vi "ALL arduinos connected 2.vi"() -> ()   [LabVIEW 2014]
uses:
  <vilib>/Utility/error.llb/DialogType.ctl
  <vilib>/Analysis/baseanly.llb/Mean (DBL).vi
  <vilib>/Instr/_visa.llb/VISA Configure Serial Port (Instr).vi
  <vilib>/Utility/file.llb/Write To Spreadsheet File (string).vi
  <vilib>/Utility/file.llb/Write To Spreadsheet File (DBL).vi
  <vilib>/Analysis/NI_AALBase.lvlib
panel:
  out "Input 6":string
  out "X 6":dbl format="%#_8g"
  out "x-y 6":dbl
  out "Y 6 7":dbl format="%#_8g"
  out "Waveform Chart 20":dbl[](graph) caption="Waveform Chart"
  out "Frequency 6":dbl format="%#_8g"
  out "Waveform Chart 19":dbl(graph) caption="Waveform Chart"
  out "Temperature 6":dbl
  out "Median 6":dbl format="%0.2f"
  out "Mean 6":dbl format="%0.2f"
  out "Waveform Chart 18":dbl(graph) caption="Waveform Chart"
  out "Input 5":string
  out "X 5":dbl format="%#_8g"
  out "x-y 5":dbl
  out "Y 5":dbl format="%#_8g"
  out "Waveform Chart 17":dbl[](graph) caption="Waveform Chart"
  out "Frequency 5":dbl format="%#_8g"
  out "Waveform Chart 16":dbl(graph) caption="Waveform Chart"
  out "Temperature 5":dbl
  out "Median 5":dbl format="%0.2f"
  out "Mean 5":dbl format="%0.2f"
  out "Waveform Chart 15":dbl(graph) caption="Waveform Chart"
  out "Input 4":string
  out "X 4":dbl format="%#_8g"
  out "x-y 4":dbl
  out "Y 4":dbl format="%#_8g"
  out "Waveform Chart 14":dbl[](graph) caption="Waveform Chart"
  out "Frequency 4":dbl format="%#_8g"
  out "Waveform Chart 6":dbl(graph) caption="Waveform Chart"
  out "Temperature 5":dbl
  out "Median 4":dbl format="%0.2f"
  out "Mean 4":dbl format="%0.2f"
  out "Waveform Chart 13":dbl(graph) caption="Waveform Chart"
  out "Input  3":string
  out "X 3":dbl format="%#_8g"
  out "x-y 3":dbl
  out "Y 3":dbl format="%#_8g"
  out "Waveform Chart 12":dbl[](graph) caption="Waveform Chart"
  out "Frequency 3":dbl format="%#_8g"
  out "Waveform Chart 5":dbl(graph) caption="Waveform Chart"
  out "Temperature 3":dbl
  out "Median 3":dbl format="%0.2f"
  out "Mean 3":dbl format="%0.2f"
  out "Waveform Chart 11":dbl(graph) caption="Waveform Chart"
  out "Input 1":string
  out "Input 2":string
  out "X 2":dbl format="%#_8g"
  out "x-y 2":dbl
  out "Y 2":dbl format="%#_8g"
  out "Waveform Chart 10":dbl[](graph) caption="Waveform Chart"
  out "Frequency 2":dbl format="%#_8g"
  out "Waveform Chart 4":dbl(graph) caption="Waveform Chart"
  out "Temperature 2":dbl
  out "Median 2":dbl format="%0.2f"
  out "Mean 2":dbl format="%0.2f"
  out "Waveform Chart 9":dbl(graph) caption="Waveform Chart"
  out "X 1 2":dbl format="%#_8g"
  out "x-y 1":dbl
  out "Y 1":dbl format="%#_8g"
  out "Waveform Chart 8":dbl[](graph) caption="Waveform Chart"
  out "Frequency 1":dbl format="%#_8g"
  out "Waveform Chart 3":dbl(graph) caption="Waveform Chart"
  out "Temperature 1":dbl
  out "Waveform Chart 7":dbl(graph) caption="Waveform Chart"
  out "Mean":dbl format="%0.2f"
  out "Median":dbl format="%0.2f"
  in  "STOP":bool
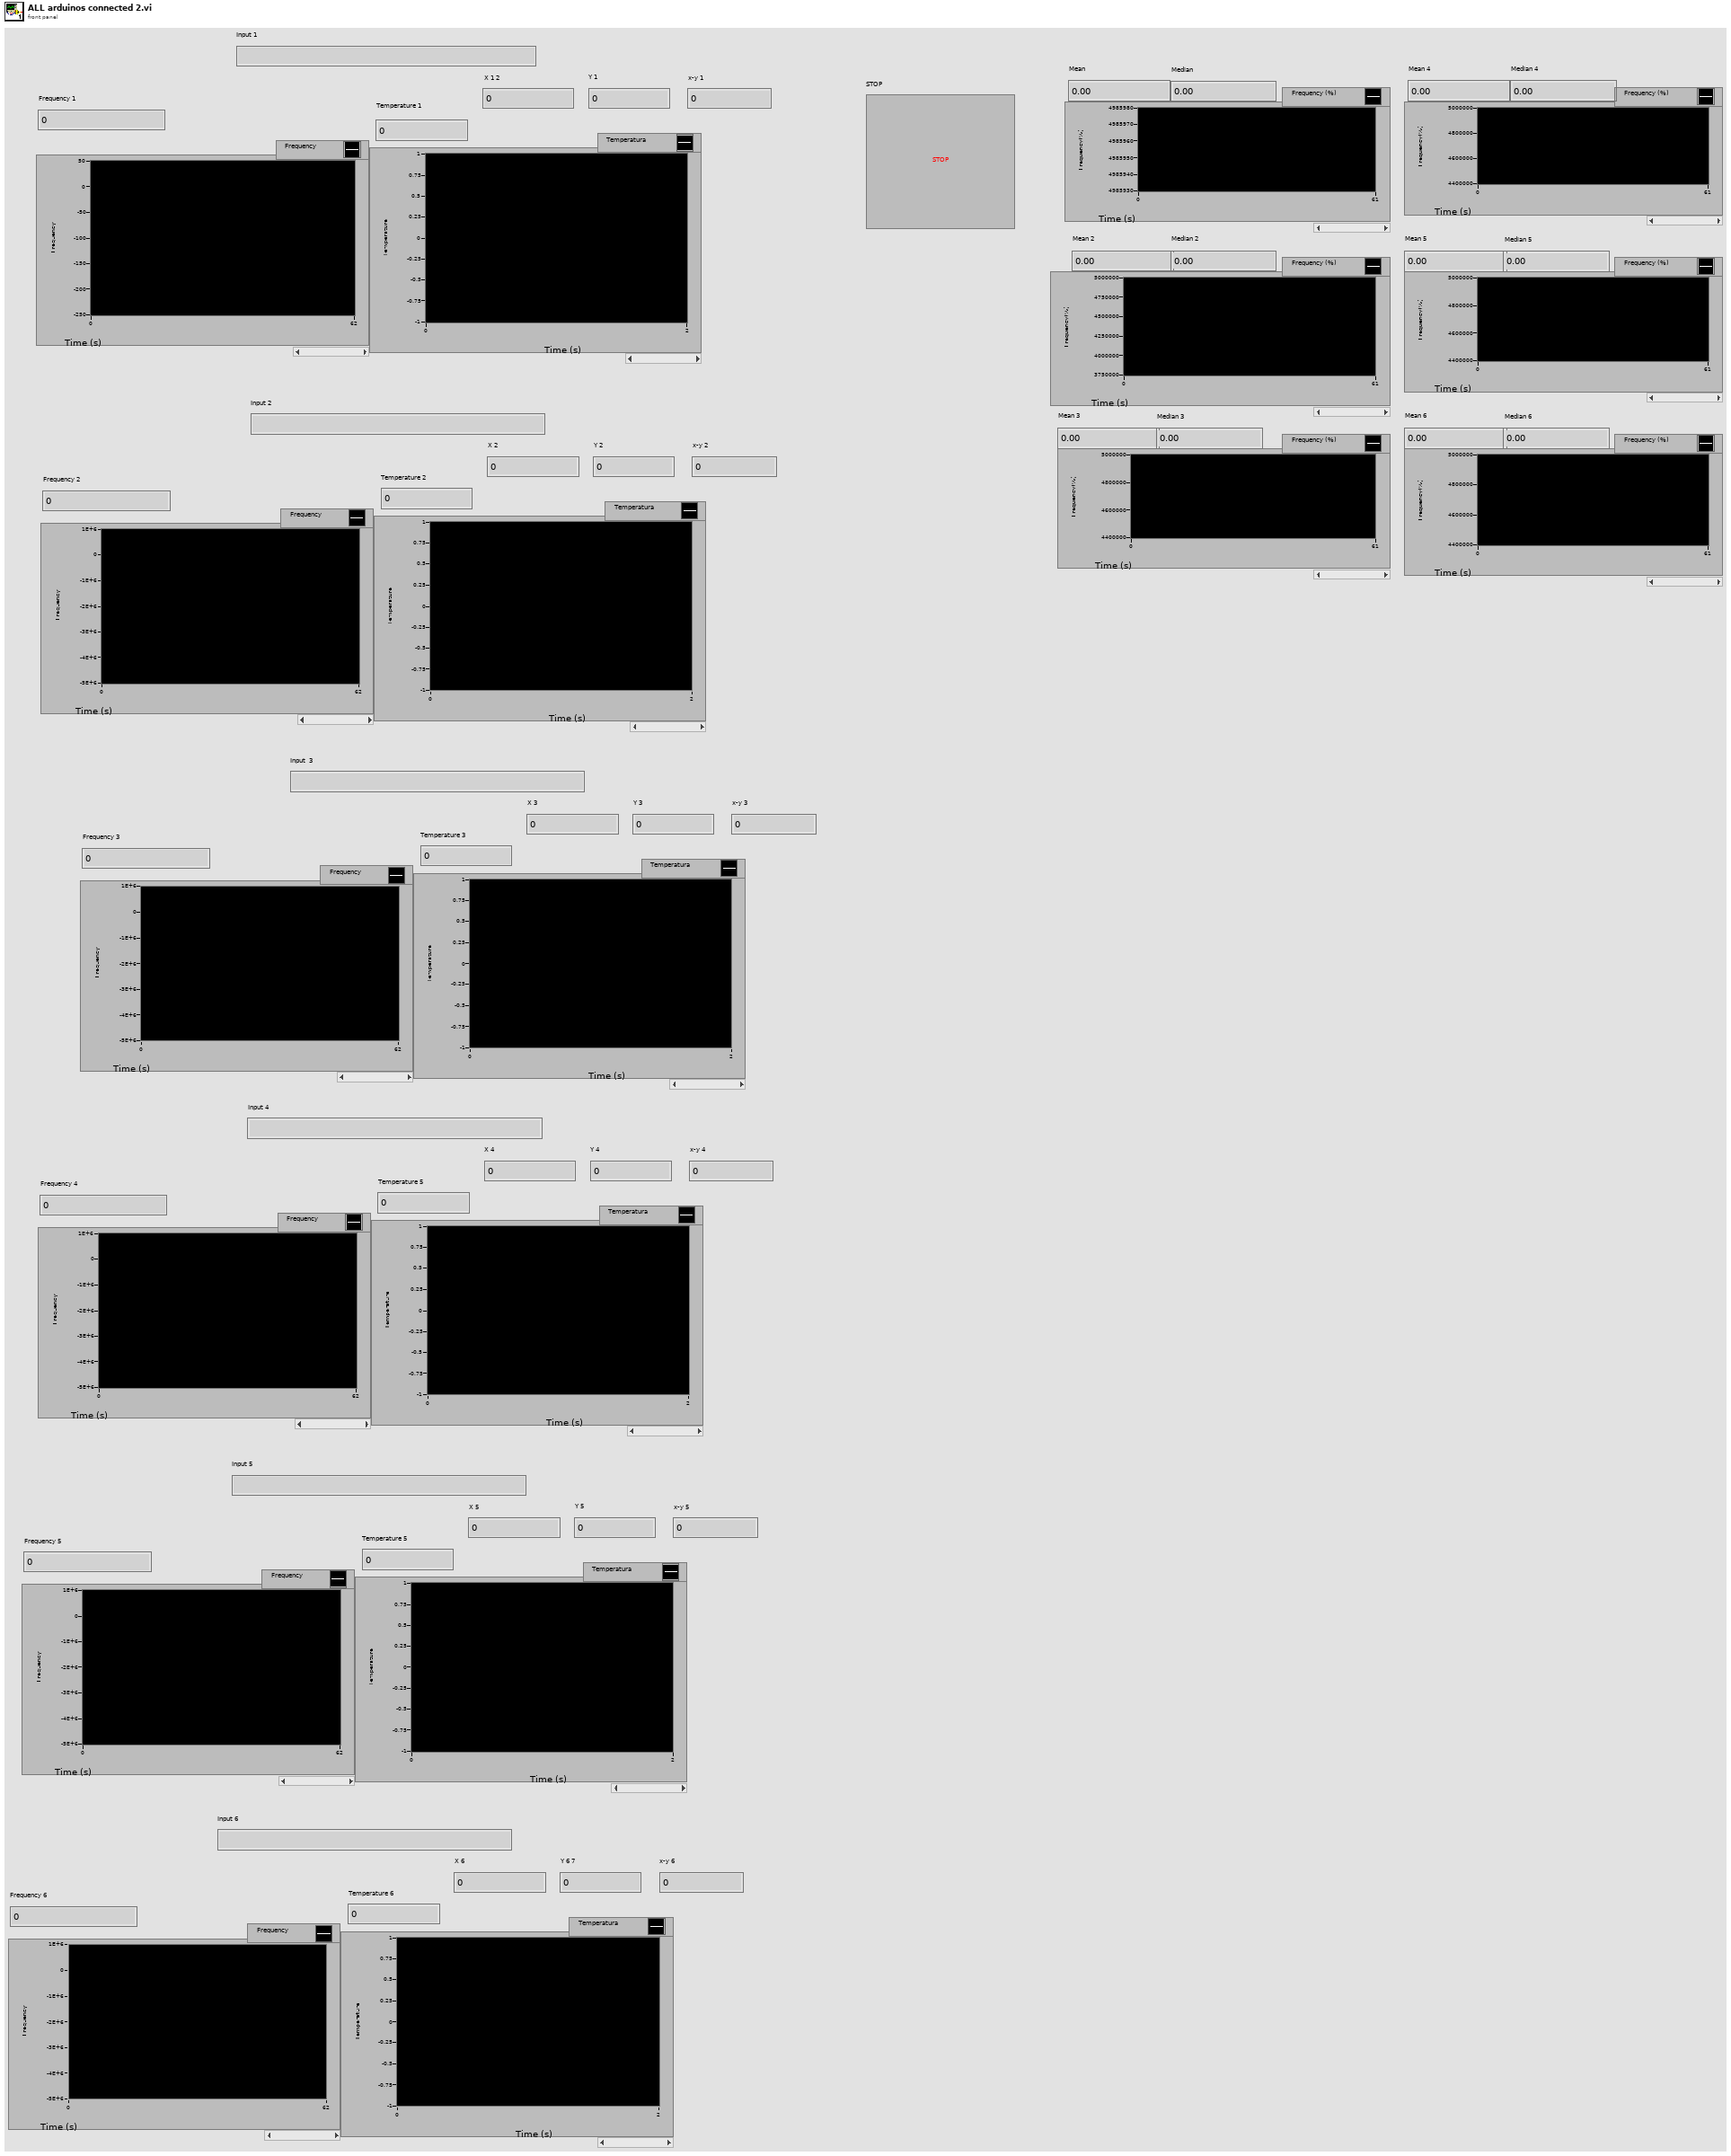
[diagram p1: front panel]
types:
  T1 = typedef "DialogType.ctl" = u16
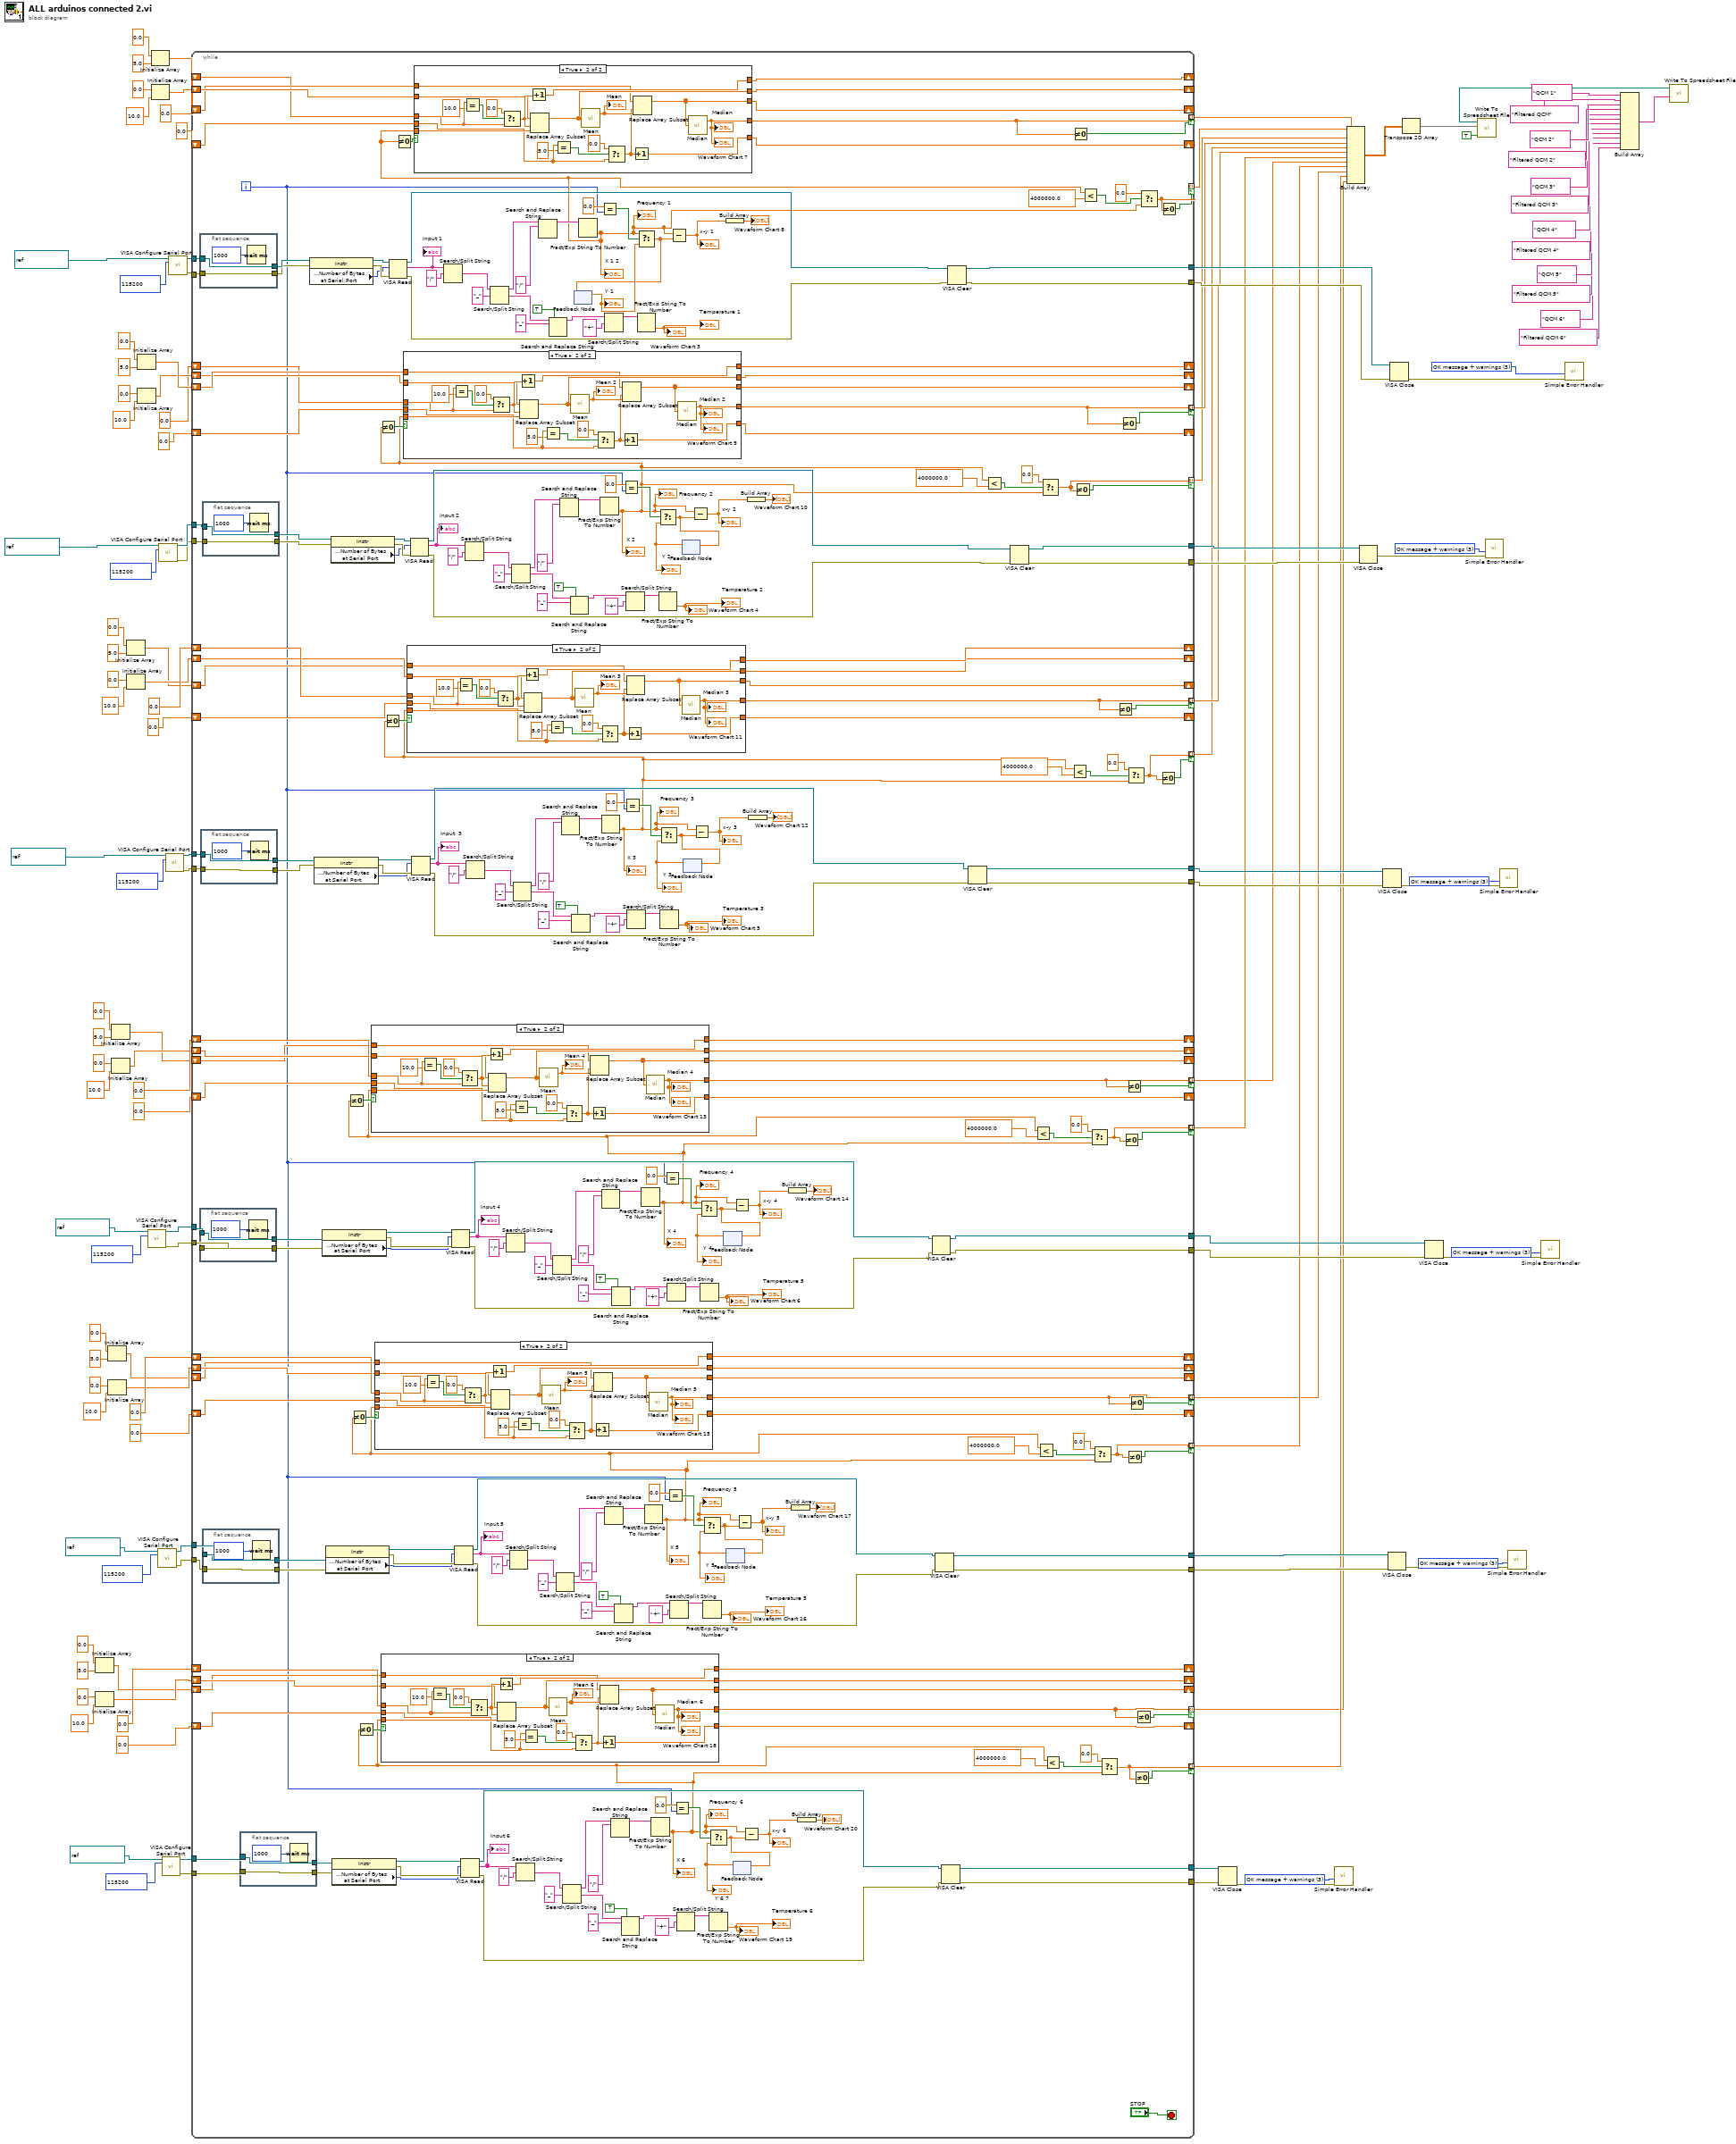
[diagram p0: block diagram]
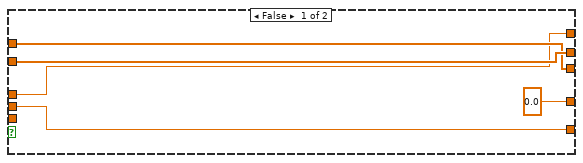
[diagram p2: hidden frame]
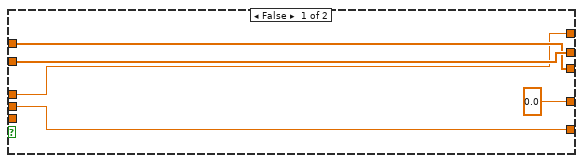
[diagram p3: hidden frame]
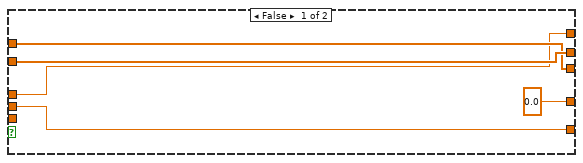
[diagram p4: hidden frame]
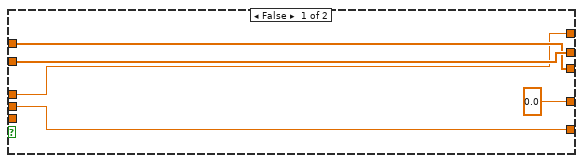
[diagram p5: hidden frame]
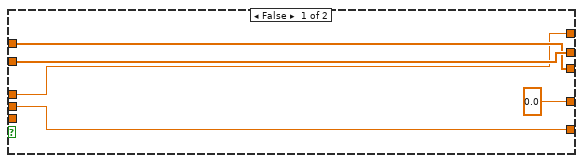
[diagram p6: hidden frame]
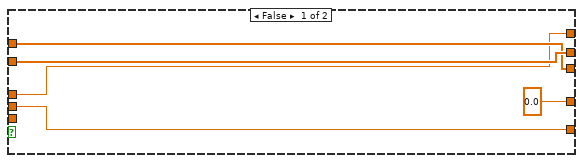
[diagram p7: hidden frame]
diagram:
  w6 = T1 3 items=["no dialog", "OK message", "continue or stop message", "OK message + warnings", "continue/stop + warnings"] ("type of dialog (OK msg:1)")
  w32 = T1 3 items=["no dialog", "OK message", "continue or stop message", "OK message + warnings", "continue/stop + warnings"] ("type of dialog (OK msg:1)")
  w48 = T1 3 items=["no dialog", "OK message", "continue or stop message", "OK message + warnings", "continue/stop + warnings"] ("type of dialog (OK msg:1)")
  w67 = T1 3 items=["no dialog", "OK message", "continue or stop message", "OK message + warnings", "continue/stop + warnings"] ("type of dialog (OK msg:1)")
  w90 = T1 3 items=["no dialog", "OK message", "continue or stop message", "OK message + warnings", "continue/stop + warnings"] ("type of dialog (OK msg:1)")
  w106 = T1 3 items=["no dialog", "OK message", "continue or stop message", "OK message + warnings", "continue/stop + warnings"] ("type of dialog (OK msg:1)")
  n1 = Initialize Array(0.0 ("x"), 5.0 ("x")) -> (w12:dbl[])
  n2 = Initialize Array(0.0 ("x"), 10.0 ("x")) -> (w13:dbl[])
  n3 = Initialize Array(0.0 ("x"), 5.0 ("x")) -> (w34:dbl[])
  n4 = Initialize Array(0.0 ("x"), 10.0 ("x")) -> (w35:dbl[])
  n5 = Initialize Array(0.0 ("x"), 5.0 ("x")) -> (w54:dbl[])
  n6 = Initialize Array(0.0 ("x"), 10.0 ("x")) -> (w55:dbl[])
  n7 = Initialize Array(0.0 ("x"), 5.0 ("x")) -> (w73:dbl[])
  n8 = Initialize Array(0.0 ("x"), 10.0 ("x")) -> (w74:dbl[])
  n9 = Initialize Array(0.0 ("x"), 5.0 ("x")) -> (w83:dbl[])
  n10 = Initialize Array(0.0 ("x"), 10.0 ("x")) -> (w82:dbl[])
  n11 = call-poly "VISA Configure Serial Port"("VISA resource name"=refnum<visa-resource-name> "COM12", "baud rate (9600)"=u32 115200) -> ("VISA resource name out"=w50:refnum<visa-resource-name>, "error out"=w49:errorcluster)  [unwired: 12 in]
  n12 = Initialize Array(0.0 ("x"), 5.0 ("x")) -> (w115:dbl[])
  n13 = Initialize Array(0.0 ("x"), 10.0 ("x")) -> (w119:dbl[])
  n14 = call-poly "VISA Configure Serial Port"("VISA resource name"=refnum<visa-resource-name> "COM12", "baud rate (9600)"=u32 115200) -> ("VISA resource name out"=w20:refnum<visa-resource-name>, "error out"=w19:errorcluster)  [unwired: 12 in]
  n15 = call-poly "VISA Configure Serial Port"("VISA resource name"=refnum<visa-resource-name> "COM12", "baud rate (9600)"=u32 115200) -> ("VISA resource name out"=w92:refnum<visa-resource-name>, "error out"=w91:errorcluster)  [unwired: 12 in]
  n16 = call-poly "VISA Configure Serial Port"("VISA resource name"=refnum<visa-resource-name> "COM12", "baud rate (9600)"=u32 115200) -> ("VISA resource name out"=w8:refnum<visa-resource-name>, "error out"=w7:errorcluster)  [unwired: 12 in]
  n17 = call-poly "VISA Configure Serial Port"("VISA resource name"=refnum<visa-resource-name> "COM12", "baud rate (9600)"=u32 115200) -> ("VISA resource name out"=w69:refnum<visa-resource-name>, "error out"=w68:errorcluster)  [unwired: 12 in]
  n18 = call-poly "VISA Configure Serial Port"("VISA resource name"=refnum<visa-resource-name> "COM10", "baud rate (9600)"=u32 115200) -> ("VISA resource name out"=w108:refnum<visa-resource-name>, "error out"=w107:errorcluster)  [unwired: 12 in]
  n19 = while {
    shift-right: [w369] -> _
    shift-left: w119 -> [w414]
    shift-right: [w368] -> _
    shift-left: 0.0 ("x") -> [w327]
    shift-right: [w412] -> _
    shift-left: w115 -> [w411]
    shift-right: [w410] -> _
    shift-left: 0.0 ("x") -> [w409]
    tunnel: [w407] -> w85 mode=indexing if=w408
    tunnel: w108 -> [w406]
    tunnel: w107 -> [w405]
    tunnel: [w377] -> w104
    tunnel: [w376] -> w103
    tunnel: [w372] -> w86 mode=indexing if=w371
    tunnel: [w366] -> w84 mode=indexing if=w367
    tunnel: w92 -> [w339]
    tunnel: w91 -> [w338]
    tunnel: [w333] -> w88
    tunnel: [w332] -> w87
    tunnel: [w331] -> w63 mode=indexing if=w330
    shift-right: [w326] -> _
    shift-left: w83 -> [w325]
    shift-right: [w323] -> _
    shift-left: w82 -> [w324]
    shift-right: [w321] -> _
    shift-left: 0.0 ("x") -> [w322]
    shift-right: [w319] -> _
    shift-left: 0.0 ("x") -> [w320]
    tunnel: [w308] -> w62 mode=indexing if=w309
    shift-right: [w313] -> _
    shift-left: 0.0 ("x") -> [w317]
    shift-right: [w312] -> _
    shift-left: w74 -> [w316]
    shift-right: [w311] -> _
    shift-left: w73 -> [w315]
    shift-right: [w310] -> _
    shift-left: 0.0 ("x") -> [w314]
    tunnel: w69 -> [w307]
    tunnel: w68 -> [w306]
    tunnel: [w278] -> w65
    tunnel: [w277] -> w64
    tunnel: [w272] -> w61 mode=indexing if=w271
    tunnel: w50 -> [w265]
    tunnel: w49 -> [w264]
    tunnel: [w236] -> w46
    tunnel: [w235] -> w45
    tunnel: [w231] -> w42 mode=indexing if=w230
    shift-right: [w228] -> _
    shift-left: 0.0 ("x") -> [w269]
    shift-right: [w227] -> _
    shift-left: w55 -> [w268]
    shift-right: [w226] -> _
    shift-left: w54 -> [w267]
    tunnel: [w224] -> w41 mode=indexing if=w225
    shift-right: [w223] -> _
    shift-left: 0.0 ("x") -> [w266]
    tunnel: [w186] -> w26 mode=indexing if=w185
    tunnel: [w181] -> w25 mode=indexing if=w180
    shift-right: [w184] -> _
    shift-left: 0.0 ("x") -> [w190]
    shift-right: [w183] -> _
    shift-left: w35 -> [w189]
    shift-right: [w182] -> _
    shift-left: w34 -> [w188]
    shift-right: [w179] -> _
    shift-left: 0.0 ("x") -> [w187]
    tunnel: [w178] -> w30
    tunnel: [w177] -> w29
    tunnel: w20 -> [w145]
    tunnel: w19 -> [w144]
    tunnel: w8 -> [w138]
    tunnel: w7 -> [w137]
    tunnel: [w132] -> w1 mode=indexing if=w131
    tunnel: [w129] -> w2 mode=indexing if=w128
    tunnel: [w127] -> w4
    tunnel: [w126] -> w3
    shift-right: [w135] -> _
    shift-left: 0.0 ("x") -> [w143]
    shift-right: [w134] -> _
    shift-left: w13 -> [w142]
    shift-right: [w133] -> _
    shift-left: w12 -> [w141]
    shift-right: [w130] -> _
    shift-left: 0.0 ("x") -> [w140]
    i -> [w139]
    stop <- "STOP" stop-if-true
    n20 = flat-sequence {
      tunnel: [w471] -> w262
      tunnel: w265 -> [w471]
      tunnel: w264 -> [w470]
      tunnel: [w470] -> w263
      frame #0 {
        n21 = Wait (ms)(milliseconds to wait=u32 1000) -> ()  [unwired: 1 out]
      }
    }
    n22 = flat-sequence {
      tunnel: [w552] -> w381
      tunnel: w406 -> [w552]
      tunnel: w405 -> [w551]
      tunnel: [w551] -> w380
      frame #0 {
        n23 = Wait (ms)(milliseconds to wait=u32 1000) -> ()  [unwired: 1 out]
      }
    }
    n24 = flat-sequence {
      tunnel: [w498] -> w282
      tunnel: w307 -> [w498]
      tunnel: w306 -> [w497]
      tunnel: [w497] -> w281
      frame #0 {
        n25 = Wait (ms)(milliseconds to wait=u32 1000) -> ()  [unwired: 1 out]
      }
    }
    n26 = flat-sequence {
      tunnel: [w525] -> w337
      tunnel: w339 -> [w525]
      tunnel: w338 -> [w524]
      tunnel: [w524] -> w336
      frame #0 {
        n27 = Wait (ms)(milliseconds to wait=u32 1000) -> ()  [unwired: 1 out]
      }
    }
    n28 = flat-sequence {
      tunnel: [w444] -> w220
      tunnel: w145 -> [w444]
      tunnel: w144 -> [w443]
      tunnel: [w443] -> w221
      frame #0 {
        n29 = Wait (ms)(milliseconds to wait=u32 1000) -> ()  [unwired: 1 out]
      }
    }
    n30 = flat-sequence {
      tunnel: [w417] -> w174
      tunnel: w138 -> [w417]
      tunnel: w137 -> [w416]
      tunnel: [w416] -> w175
      frame #0 {
        n31 = Wait (ms)(milliseconds to wait=u32 1000) -> ()  [unwired: 1 out]
      }
    }
    n32 = property class="Instr"(reference=w381, error in=w380) -> (reference out=w385:refnum<visa-resource-name>, error out=w384:errorcluster, "Serial Settings:Number of Bytes at Serial Port"=w383:u32)
    n33 = property class="Instr"(reference=w282, error in=w281) -> (reference out=w286:refnum<visa-resource-name>, error out=w285:errorcluster, "Serial Settings:Number of Bytes at Serial Port"=w284:u32)
    n34 = property class="Instr"(reference=w262, error in=w263) -> (reference out=w241:refnum<visa-resource-name>, error out=w240:errorcluster, "Serial Settings:Number of Bytes at Serial Port"=w239:u32)
    n35 = property class="Instr"(reference=w220, error in=w221) -> (reference out=w199:refnum<visa-resource-name>, error out=w198:errorcluster, "Serial Settings:Number of Bytes at Serial Port"=w197:u32)
    n36 = property class="Instr"(reference=w337, error in=w336) -> (reference out=w343:refnum<visa-resource-name>, error out=w342:errorcluster, "Serial Settings:Number of Bytes at Serial Port"=w341:u32)
    n37 = property class="Instr"(reference=w174, error in=w175) -> (reference out=w153:refnum<visa-resource-name>, error out=w152:errorcluster, "Serial Settings:Number of Bytes at Serial Port"=w151:u32)
    n38 = VISA Read(VISA resource name=w385, byte count=w383, error in (no error)=w384) -> (VISA resource name out=w378:refnum<visa-resource-name>, read buffer=w386:string, error out=w379:errorcluster)  [unwired: 1 out]
    "Input 1" <- w386
    n39 = VISA Read(VISA resource name=w343, byte count=w341, error in (no error)=w342) -> (VISA resource name out=w335:refnum<visa-resource-name>, read buffer=w344:string, error out=w334:errorcluster)  [unwired: 1 out]
    "Input 2" <- w344
    n40 = VISA Read(VISA resource name=w286, byte count=w284, error in (no error)=w285) -> (VISA resource name out=w280:refnum<visa-resource-name>, read buffer=w287:string, error out=w279:errorcluster)  [unwired: 1 out]
    "Input  3" <- w287
    n41 = Search/Split String(string=w386, search string/char (-)="/") -> (match + rest of string=w395:string)  [unwired: 1 in, 2 out]
    n42 = VISA Read(VISA resource name=w241, byte count=w239, error in (no error)=w240) -> (VISA resource name out=w238:refnum<visa-resource-name>, read buffer=w243:string, error out=w237:errorcluster)  [unwired: 1 out]
    "Input 4" <- w243
    n43 = VISA Read(VISA resource name=w199, byte count=w197, error in (no error)=w198) -> (VISA resource name out=w196:refnum<visa-resource-name>, read buffer=w201:string, error out=w195:errorcluster)  [unwired: 1 out]
    "Input 5" <- w201
    n44 = VISA Read(VISA resource name=w153, byte count=w151, error in (no error)=w152) -> (VISA resource name out=w150:refnum<visa-resource-name>, read buffer=w155:string, error out=w136:errorcluster)  [unwired: 1 out]
    "Input 6" <- w155
    n45 = Search/Split String(string=w344, search string/char (-)="/") -> (match + rest of string=w353:string)  [unwired: 1 in, 2 out]
    n46 = Search/Split String(string=w287, search string/char (-)="/") -> (match + rest of string=w296:string)  [unwired: 1 in, 2 out]
    n47 = Search/Split String(string=w395, search string/char (-)="_") -> (substring before match=w388:string, match + rest of string=w394:string)  [unwired: 1 in, 1 out]
    n48 = Search/Split String(string=w243, search string/char (-)="/") -> (match + rest of string=w252:string)  [unwired: 1 in, 2 out]
    n49 = Search/Split String(string=w201, search string/char (-)="/") -> (match + rest of string=w210:string)  [unwired: 1 in, 2 out]
    n50 = Search/Split String(string=w353, search string/char (-)="_") -> (substring before match=w346:string, match + rest of string=w352:string)  [unwired: 1 in, 1 out]
    n51 = Search/Split String(string=w296, search string/char (-)="_") -> (substring before match=w289:string, match + rest of string=w295:string)  [unwired: 1 in, 1 out]
    n52 = Search/Split String(string=w155, search string/char (-)="/") -> (match + rest of string=w164:string)  [unwired: 1 in, 2 out]
    n53 = Search and Replace String(input string=w388, search string="/" ("replace string (\"\")")) -> (result string=w398:string)  [unwired: 6 in, 3 out]
    n54 = Search and Replace String(replace all?=TRUE ("replace all? (F)"), input string=w394, search string="_") -> (result string=w390:string)  [unwired: 5 in, 3 out]
    n55 = Search/Split String(string=w252, search string/char (-)="_") -> (substring before match=w245:string, match + rest of string=w251:string)  [unwired: 1 in, 1 out]
    n56 = Search/Split String(string=w210, search string/char (-)="_") -> (substring before match=w203:string, match + rest of string=w209:string)  [unwired: 1 in, 1 out]
    n57 = Search and Replace String(input string=w346, search string="/" ("replace string (\"\")")) -> (result string=w356:string)  [unwired: 6 in, 3 out]
    n58 = Search and Replace String(input string=w289, search string="/" ("replace string (\"\")")) -> (result string=w299:string)  [unwired: 6 in, 3 out]
    n59 = Search/Split String(string=w164, search string/char (-)="_") -> (substring before match=w157:string, match + rest of string=w163:string)  [unwired: 1 in, 1 out]
    n60 = Search and Replace String(replace all?=TRUE ("replace all? (F)"), input string=w352, search string="_") -> (result string=w348:string)  [unwired: 5 in, 3 out]
    n61 = Search and Replace String(replace all?=TRUE ("replace all? (F)"), input string=w295, search string="_") -> (result string=w291:string)  [unwired: 5 in, 3 out]
    n62 = feedback #1() -> (w402:dbl)  [unwired: 1 in]
    "Y 1" <- w402
    n63 = Fract/Exp String To Number(string=w398) -> (number=w370:dbl)  [unwired: 3 in, 1 out]
    "Frequency 1" <- w370
    "X 1 2" <- w370
    n64 = Not Equal To 0?(x=w370) -> (x != 0?=w413:bool)
    n65 = case shown="True" w413 {
      tunnel: w414 -> [w558 w571]
      tunnel: w327 -> [w555 w574]
      tunnel: [w555 w573] -> w368
      tunnel: w370 -> [_ w572]
      tunnel: [w558 w570] -> w369
      tunnel: [w557 w562] -> w412
      tunnel: w411 -> [w557 w563]
      tunnel: w409 -> [w556 w566]
      tunnel: [w556 w564] -> w410
      tunnel: [0.0 ("median") w559] -> w407
      frame False {
      }
      frame True {
        n66 = Equal?(x=w574, y=10.0) -> (x = y?=w577:bool)
        n67 = Select(t=0.0, s=w577, f=w574) -> (s? t:f=w575:dbl)
        n68 = Increment(x=w575) -> (x+1=w573:dbl)
        n69 = Replace Array Subset(array=w571, new element=w572, index=w575) -> (w570:dbl[])
        n70 = Equal?(x=w566, y=5.0) -> (x = y?=w567:bool)
        n71 = call-poly <vilib>:"Mean.vi"("X"=w570) -> ("mean"=w569:dbl)  [unwired: 1 out]
        "Mean" <- w569
        n72 = Select(t=0.0, s=w567, f=w566) -> (s? t:f=w565:dbl)
        n73 = Increment(x=w565) -> (x+1=w564:dbl)
        n74 = Replace Array Subset(array=w563, new element=w569, index=w565) -> (w562:dbl[])
        n75 = call <vilib>:"Median.vi"("X"=w562) -> ("median"=w559:dbl)  [unwired: 1 out]
        "Median" <- w559
        "Waveform Chart 7" <- w559
      }
    }
    n76 = Fract/Exp String To Number(string=w356) -> (number=w328:dbl)  [unwired: 3 in, 1 out]
    "Frequency 2" <- w328
    "X 2" <- w328
    n77 = Not Equal To 0?(x=w328) -> (x != 0?=w329:bool)
    n78 = case shown="True" w329 {
      tunnel: w324 -> [w531 w544]
      tunnel: w322 -> [w528 w547]
      tunnel: [w528 w546] -> w321
      tunnel: w328 -> [_ w545]
      tunnel: [w531 w543] -> w323
      tunnel: [w530 w535] -> w326
      tunnel: w325 -> [w530 w536]
      tunnel: w320 -> [w529 w539]
      tunnel: [w529 w537] -> w319
      tunnel: [0.0 ("median") w532] -> w366
      frame False {
      }
      frame True {
        n79 = Equal?(x=w547, y=10.0) -> (x = y?=w550:bool)
        n80 = Select(t=0.0, s=w550, f=w547) -> (s? t:f=w548:dbl)
        n81 = Increment(x=w548) -> (x+1=w546:dbl)
        n82 = Replace Array Subset(array=w544, new element=w545, index=w548) -> (w543:dbl[])
        n83 = Equal?(x=w539, y=5.0) -> (x = y?=w540:bool)
        n84 = call-poly <vilib>:"Mean.vi"("X"=w543) -> ("mean"=w542:dbl)  [unwired: 1 out]
        "Mean 2" <- w542
        n85 = Select(t=0.0, s=w540, f=w539) -> (s? t:f=w538:dbl)
        n86 = Increment(x=w538) -> (x+1=w537:dbl)
        n87 = Replace Array Subset(array=w536, new element=w542, index=w538) -> (w535:dbl[])
        n88 = call <vilib>:"Median.vi"("X"=w535) -> ("median"=w532:dbl)  [unwired: 1 out]
        "Median 2" <- w532
        "Waveform Chart 9" <- w532
      }
    }
    n89 = Equal?(x=0.0, y=w139) -> (x = y?=w403:bool)
    n90 = Fract/Exp String To Number(string=w299) -> (number=w273:dbl)  [unwired: 3 in, 1 out]
    "Frequency 3" <- w273
    "X 3" <- w273
    n91 = Not Equal To 0?(x=w273) -> (x != 0?=w318:bool)
    n92 = case shown="True" w318 {
      tunnel: w316 -> [w504 w517]
      tunnel: w317 -> [w501 w520]
      tunnel: [w501 w519] -> w313
      tunnel: w273 -> [_ w518]
      tunnel: [w504 w516] -> w312
      tunnel: [w503 w508] -> w311
      tunnel: w315 -> [w503 w509]
      tunnel: w314 -> [w502 w512]
      tunnel: [w502 w510] -> w310
      tunnel: [0.0 ("median") w505] -> w308
      frame False {
      }
      frame True {
        n93 = Equal?(x=w520, y=10.0) -> (x = y?=w523:bool)
        n94 = Select(t=0.0, s=w523, f=w520) -> (s? t:f=w521:dbl)
        n95 = Increment(x=w521) -> (x+1=w519:dbl)
        n96 = Replace Array Subset(array=w517, new element=w518, index=w521) -> (w516:dbl[])
        n97 = Equal?(x=w512, y=5.0) -> (x = y?=w513:bool)
        n98 = call-poly <vilib>:"Mean.vi"("X"=w516) -> ("mean"=w515:dbl)  [unwired: 1 out]
        "Mean 3" <- w515
        n99 = Select(t=0.0, s=w513, f=w512) -> (s? t:f=w511:dbl)
        n100 = Increment(x=w511) -> (x+1=w510:dbl)
        n101 = Replace Array Subset(array=w509, new element=w515, index=w511) -> (w508:dbl[])
        n102 = call <vilib>:"Median.vi"("X"=w508) -> ("median"=w505:dbl)  [unwired: 1 out]
        "Median 3" <- w505
        "Waveform Chart 11" <- w505
      }
    }
    n103 = Search and Replace String(input string=w245, search string="/" ("replace string (\"\")")) -> (result string=w255:string)  [unwired: 6 in, 3 out]
    n104 = Search/Split String(string=w390, search string/char (-)="+") -> (substring before match=w391:string)  [unwired: 1 in, 2 out]
    n105 = Search and Replace String(input string=w203, search string="/" ("replace string (\"\")")) -> (result string=w213:string)  [unwired: 6 in, 3 out]
    n106 = Search and Replace String(input string=w157, search string="/" ("replace string (\"\")")) -> (result string=w167:string)  [unwired: 6 in, 3 out]
    n107 = Search and Replace String(replace all?=TRUE ("replace all? (F)"), input string=w251, search string="_") -> (result string=w247:string)  [unwired: 5 in, 3 out]
    n108 = Search and Replace String(replace all?=TRUE ("replace all? (F)"), input string=w209, search string="_") -> (result string=w205:string)  [unwired: 5 in, 3 out]
    n109 = Search and Replace String(replace all?=TRUE ("replace all? (F)"), input string=w163, search string="_") -> (result string=w159:string)  [unwired: 5 in, 3 out]
    n110 = Equal?(x=0.0, y=w139) -> (x = y?=w361:bool)
    n111 = Equal?(x=0.0, y=w139) -> (x = y?=w304:bool)
    n112 = Search/Split String(string=w348, search string/char (-)="+") -> (substring before match=w349:string)  [unwired: 1 in, 2 out]
    n113 = Search/Split String(string=w291, search string/char (-)="+") -> (substring before match=w292:string)  [unwired: 1 in, 2 out]
    n114 = Select(t=w370, s=w403, f=w402) -> (s? t:f=w401:dbl)
    n115 = feedback-in #1(w401) -> ()
    n116 = Fract/Exp String To Number(string=w391) -> (number=→"Temperature 1" →"Waveform Chart 3":dbl)  [unwired: 3 in, 1 out]
    n117 = Fract/Exp String To Number(string=w255) -> (number=w229:dbl)  [unwired: 3 in, 1 out]
    "Frequency 4" <- w229
    "X 4" <- w229
    n118 = Not Equal To 0?(x=w229) -> (x != 0?=w270:bool)
    n119 = case shown="True" w270 {
      tunnel: w268 -> [w477 w490]
      tunnel: w269 -> [w474 w493]
      tunnel: [w474 w492] -> w228
      tunnel: w229 -> [_ w491]
      tunnel: [w477 w489] -> w227
      tunnel: [w476 w482] -> w226
      tunnel: w267 -> [w476 w483]
      tunnel: w266 -> [w475 w478]
      tunnel: [w475 w484] -> w223
      tunnel: [0.0 ("median") w479] -> w224
      frame False {
      }
      frame True {
        n120 = Equal?(x=w493, y=10.0) -> (x = y?=w496:bool)
        n121 = Select(t=0.0, s=w496, f=w493) -> (s? t:f=w494:dbl)
        n122 = Increment(x=w494) -> (x+1=w492:dbl)
        n123 = Replace Array Subset(array=w490, new element=w491, index=w494) -> (w489:dbl[])
        n124 = Equal?(x=w478, y=5.0) -> (x = y?=w486:bool)
        n125 = call-poly <vilib>:"Mean.vi"("X"=w489) -> ("mean"=w488:dbl)  [unwired: 1 out]
        "Mean 4" <- w488
        n126 = Select(t=0.0, s=w486, f=w478) -> (s? t:f=w485:dbl)
        n127 = Increment(x=w485) -> (x+1=w484:dbl)
        n128 = Replace Array Subset(array=w483, new element=w488, index=w485) -> (w482:dbl[])
        n129 = call <vilib>:"Median.vi"("X"=w482) -> ("median"=w479:dbl)  [unwired: 1 out]
        "Median 4" <- w479
        "Waveform Chart 13" <- w479
      }
    }
    n130 = Fract/Exp String To Number(string=w213) -> (number=w191:dbl)  [unwired: 3 in, 1 out]
    "Frequency 5" <- w191
    "X 5" <- w191
    n131 = Not Equal To 0?(x=w191) -> (x != 0?=w222:bool)
    n132 = case shown="True" w222 {
      tunnel: w189 -> [w450 w463]
      tunnel: w190 -> [w447 w466]
      tunnel: [w447 w465] -> w184
      tunnel: w191 -> [_ w464]
      tunnel: [w450 w462] -> w183
      tunnel: [w449 w455] -> w182
      tunnel: w188 -> [w449 w456]
      tunnel: w187 -> [w448 w451]
      tunnel: [w448 w457] -> w179
      tunnel: [0.0 ("median") w452] -> w181
      frame False {
      }
      frame True {
        n133 = Equal?(x=w466, y=10.0) -> (x = y?=w469:bool)
        n134 = Select(t=0.0, s=w469, f=w466) -> (s? t:f=w467:dbl)
        n135 = Increment(x=w467) -> (x+1=w465:dbl)
        n136 = Replace Array Subset(array=w463, new element=w464, index=w467) -> (w462:dbl[])
        n137 = Equal?(x=w451, y=5.0) -> (x = y?=w459:bool)
        n138 = call-poly <vilib>:"Mean.vi"("X"=w462) -> ("mean"=w461:dbl)  [unwired: 1 out]
        "Mean 5" <- w461
        n139 = Select(t=0.0, s=w459, f=w451) -> (s? t:f=w458:dbl)
        n140 = Increment(x=w458) -> (x+1=w457:dbl)
        n141 = Replace Array Subset(array=w456, new element=w461, index=w458) -> (w455:dbl[])
        n142 = call <vilib>:"Median.vi"("X"=w455) -> ("median"=w452:dbl)  [unwired: 1 out]
        "Median 5" <- w452
        "Waveform Chart 15" <- w452
      }
    }
    n143 = Fract/Exp String To Number(string=w167) -> (number=w146:dbl)  [unwired: 3 in, 1 out]
    "Frequency 6" <- w146
    "X 6" <- w146
    n144 = Not Equal To 0?(x=w146) -> (x != 0?=w176:bool)
    n145 = case shown="True" w176 {
      tunnel: w142 -> [w423 w436]
      tunnel: w143 -> [w420 w439]
      tunnel: [w420 w438] -> w135
      tunnel: w146 -> [_ w437]
      tunnel: [w423 w435] -> w134
      tunnel: [w422 w428] -> w133
      tunnel: w141 -> [w422 w429]
      tunnel: w140 -> [w421 w424]
      tunnel: [w421 w430] -> w130
      tunnel: [0.0 ("median") w425] -> w132
      frame False {
      }
      frame True {
        n146 = Equal?(x=w439, y=10.0) -> (x = y?=w442:bool)
        n147 = Select(t=0.0, s=w442, f=w439) -> (s? t:f=w440:dbl)
        n148 = Increment(x=w440) -> (x+1=w438:dbl)
        n149 = Replace Array Subset(array=w436, new element=w437, index=w440) -> (w435:dbl[])
        n150 = Equal?(x=w424, y=5.0) -> (x = y?=w432:bool)
        n151 = call-poly <vilib>:"Mean.vi"("X"=w435) -> ("mean"=w434:dbl)  [unwired: 1 out]
        "Mean 6" <- w434
        n152 = Select(t=0.0, s=w432, f=w424) -> (s? t:f=w431:dbl)
        n153 = Increment(x=w431) -> (x+1=w430:dbl)
        n154 = Replace Array Subset(array=w429, new element=w434, index=w431) -> (w428:dbl[])
        n155 = call <vilib>:"Median.vi"("X"=w428) -> ("median"=w425:dbl)  [unwired: 1 out]
        "Median 6" <- w425
        "Waveform Chart 18" <- w425
      }
    }
    n156 = Fract/Exp String To Number(string=w349) -> (number=→"Temperature 2" →"Waveform Chart 4":dbl)  [unwired: 3 in, 1 out]
    n157 = Fract/Exp String To Number(string=w292) -> (number=→"Temperature 3" →"Waveform Chart 5":dbl)  [unwired: 3 in, 1 out]
    n158 = Equal?(x=0.0, y=w139) -> (x = y?=w260:bool)
    n159 = Equal?(x=0.0, y=w139) -> (x = y?=w218:bool)
    n160 = Search/Split String(string=w247, search string/char (-)="+") -> (substring before match=w248:string)  [unwired: 1 in, 2 out]
    n161 = Subtract(x=w370, y=w401) -> (x-y=w400:dbl)
    "x-y 1" <- w400
    n162 = Search/Split String(string=w205, search string/char (-)="+") -> (substring before match=w206:string)  [unwired: 1 in, 2 out]
    n163 = Equal?(x=0.0, y=w139) -> (x = y?=w172:bool)
    n164 = Search/Split String(string=w159, search string/char (-)="+") -> (substring before match=w160:string)  [unwired: 1 in, 2 out]
    n165 = feedback #2() -> (w360:dbl)  [unwired: 1 in]
    "Y 2" <- w360
    n166 = Select(t=w328, s=w361, f=w360) -> (s? t:f=w359:dbl)
    n167 = feedback-in #2(w359) -> ()
    n168 = feedback #3() -> (w303:dbl)  [unwired: 1 in]
    "Y 3" <- w303
    n169 = Select(t=w273, s=w304, f=w303) -> (s? t:f=w302:dbl)
    n170 = feedback-in #3(w302) -> ()
    n171 = Subtract(x=w328, y=w359) -> (x-y=w358:dbl)
    "x-y 2" <- w358
    n172 = Subtract(x=w273, y=w302) -> (x-y=w301:dbl)
    "x-y 3" <- w301
    n173 = Fract/Exp String To Number(string=w248) -> (number=→"Temperature 5" →"Waveform Chart 6":dbl)  [unwired: 3 in, 1 out]
    n174 = Fract/Exp String To Number(string=w206) -> (number=→"Temperature 5" →"Waveform Chart 16":dbl)  [unwired: 3 in, 1 out]
    n175 = Fract/Exp String To Number(string=w160) -> (number=→"Temperature 6" →"Waveform Chart 19":dbl)  [unwired: 3 in, 1 out]
    n176 = feedback #4() -> (w259:dbl)  [unwired: 1 in]
    "Y 4" <- w259
    n177 = Select(t=w229, s=w260, f=w259) -> (s? t:f=w258:dbl)
    n178 = feedback-in #4(w258) -> ()
    n179 = Build Array(w400) -> (→"Waveform Chart 8":dbl[])
    n180 = feedback #5() -> (w217:dbl)  [unwired: 1 in]
    "Y 5" <- w217
    n181 = Select(t=w191, s=w218, f=w217) -> (s? t:f=w216:dbl)
    n182 = feedback-in #5(w216) -> ()
    n183 = Subtract(x=w229, y=w258) -> (x-y=w257:dbl)
    "x-y 4" <- w257
    n184 = feedback #6() -> (w171:dbl)  [unwired: 1 in]
    "Y 6 7" <- w171
    n185 = Select(t=w146, s=w172, f=w171) -> (s? t:f=w170:dbl)
    n186 = feedback-in #6(w170) -> ()
    n187 = Subtract(x=w191, y=w216) -> (x-y=w215:dbl)
    "x-y 5" <- w215
    n188 = Subtract(x=w146, y=w170) -> (x-y=w169:dbl)
    "x-y 6" <- w169
    n189 = Build Array(w358) -> (→"Waveform Chart 10":dbl[])
    n190 = Build Array(w301) -> (→"Waveform Chart 12":dbl[])
    n191 = Build Array(w257) -> (→"Waveform Chart 14":dbl[])
    n192 = Build Array(w215) -> (→"Waveform Chart 17":dbl[])
    n193 = Build Array(w169) -> (→"Waveform Chart 20":dbl[])
    n194 = VISA Clear(VISA resource name=w238, error in (no error)=w237) -> (VISA resource name out=w236:refnum<visa-resource-name>, error out=w235:errorcluster)
    n195 = VISA Clear(VISA resource name=w196, error in (no error)=w195) -> (VISA resource name out=w178:refnum<visa-resource-name>, error out=w177:errorcluster)
    n196 = VISA Clear(VISA resource name=w150, error in (no error)=w136) -> (VISA resource name out=w127:refnum<visa-resource-name>, error out=w126:errorcluster)
    n197 = VISA Clear(VISA resource name=w378, error in (no error)=w379) -> (VISA resource name out=w377:refnum<visa-resource-name>, error out=w376:errorcluster)
    n198 = VISA Clear(VISA resource name=w280, error in (no error)=w279) -> (VISA resource name out=w278:refnum<visa-resource-name>, error out=w277:errorcluster)
    n199 = Less?(x=w328, y=4000000.0) -> (x < y?=w365:bool)
    n200 = VISA Clear(VISA resource name=w335, error in (no error)=w334) -> (VISA resource name out=w333:refnum<visa-resource-name>, error out=w332:errorcluster)
    n201 = Less?(x=w229, y=4000000.0) -> (x < y?=w234:bool)
    n202 = Less?(x=w191, y=4000000.0) -> (x < y?=w194:bool)
    n203 = Select(t=0.0, s=w365, f=w328) -> (s? t:f=w331:dbl)
    n204 = Less?(x=w146, y=4000000.0) -> (x < y?=w149:bool)
    n205 = Less?(x=w273, y=4000000.0) -> (x < y?=w276:bool)
    n206 = Not Equal To 0?(x=w407) -> (x != 0?=w408:bool)
    n207 = Not Equal To 0?(x=w331) -> (x != 0?=w330:bool)
    n208 = Less?(x=w370, y=4000000.0) -> (x < y?=w375:bool)
    n209 = Select(t=0.0, s=w234, f=w229) -> (s? t:f=w231:dbl)
    n210 = Select(t=0.0, s=w194, f=w191) -> (s? t:f=w186:dbl)
    n211 = Select(t=0.0, s=w149, f=w146) -> (s? t:f=w129:dbl)
    n212 = Not Equal To 0?(x=w308) -> (x != 0?=w309:bool)
    n213 = Not Equal To 0?(x=w366) -> (x != 0?=w367:bool)
    n214 = Not Equal To 0?(x=w231) -> (x != 0?=w230:bool)
    n215 = Not Equal To 0?(x=w224) -> (x != 0?=w225:bool)
    n216 = Not Equal To 0?(x=w186) -> (x != 0?=w185:bool)
    n217 = Select(t=0.0, s=w276, f=w273) -> (s? t:f=w272:dbl)
    n218 = Not Equal To 0?(x=w181) -> (x != 0?=w180:bool)
    n219 = Not Equal To 0?(x=w129) -> (x != 0?=w128:bool)
    n220 = Not Equal To 0?(x=w132) -> (x != 0?=w131:bool)
    n221 = Select(t=0.0, s=w375, f=w370) -> (s? t:f=w372:dbl)
    n222 = Not Equal To 0?(x=w272) -> (x != 0?=w271:bool)
    n223 = Not Equal To 0?(x=w372) -> (x != 0?=w371:bool)
  }
  n224 = VISA Close(VISA resource name=w4, error in (no error)=w3) -> (error out=w5:errorcluster)
  n225 = call <vilib>:"Simple Error Handler.vi"("type of dialog (OK msg:1)"=w6, "error in (no error)"=w5) -> ()  [unwired: 3 in, 5 out]
  n226 = Build Array(w86, w85, w63, w84, w61, w62, w42, w41, w26, w25, w2, w1) -> (w111:dbl[][])
  n227 = VISA Close(VISA resource name=w88, error in (no error)=w87) -> (error out=w89:errorcluster)
  n228 = VISA Close(VISA resource name=w65, error in (no error)=w64) -> (error out=w66:errorcluster)
  n229 = VISA Close(VISA resource name=w30, error in (no error)=w29) -> (error out=w31:errorcluster)
  n230 = VISA Close(VISA resource name=w104, error in (no error)=w103) -> (error out=w105:errorcluster)
  n231 = Transpose 2D Array(2D array=w111) -> (transposed array=w121:dbl[][])
  n232 = VISA Close(VISA resource name=w46, error in (no error)=w45) -> (error out=w47:errorcluster)
  n233 = call <vilib>:"Simple Error Handler.vi"("type of dialog (OK msg:1)"=w90, "error in (no error)"=w89) -> ()  [unwired: 3 in, 5 out]
  n234 = call <vilib>:"Simple Error Handler.vi"("type of dialog (OK msg:1)"=w67, "error in (no error)"=w66) -> ()  [unwired: 3 in, 5 out]
  n235 = call <vilib>:"Simple Error Handler.vi"("type of dialog (OK msg:1)"=w32, "error in (no error)"=w31) -> ()  [unwired: 3 in, 5 out]
  n236 = call <vilib>:"Simple Error Handler.vi"("type of dialog (OK msg:1)"=w48, "error in (no error)"=w47) -> ()  [unwired: 3 in, 5 out]
  n237 = call <vilib>:"Simple Error Handler.vi"("type of dialog (OK msg:1)"=w106, "error in (no error)"=w105) -> ()  [unwired: 3 in, 5 out]
  n238 = Build Array("QCM 1", "Filtered QCM" ("element"), "QCM 2" ("element"), "Filtered QCM 2" ("element"), "QCM 3" ("element"), "Filtered QCM 3" ("element"), "QCM 4" ("element"), "Filtered QCM 4" ("element"), "QCM 5" ("element"), "Filtered QCM 5" ("element"), "QCM 6" ("element"), "Filtered QCM 6" ("element")) -> (w123:string[])
  n239 = call-poly <vilib>:"Write To Spreadsheet File.vi"("1D data"=w123) -> ("new file path (Not A Path if cancelled)"=w124:path)  [unwired: 7 in]
  n240 = call-poly <vilib>:"Write To Spreadsheet File.vi"("append to file? (new file:F)"=TRUE, "2D data"=w121, "file path (dialog if empty)"=w124) -> ()  [unwired: 5 in, 1 out]
